vi "3Act Helper - DynamixelPositionAdjustment 0_360.vi"(10 "Dynamixel Setpoint In (deg)":dbl, 11 "Dynamixel Set Data":T1) -> (3 "Dynamixel Setpoint Out (deg)":dbl)   [LabVIEW 2013]
doc: "Because the Dynamixel is (theoretically) a 0-360 deg position controlled motor, we will need to only command 0-360 values, and keep track of the loop counts to find out where the motor really is. This really needs to be tested with the actual Dynamixels.\n\nEric Schneider, March 2014"
uses:
  Data/TypeDefs/DynamixelSetupInfo.ctl
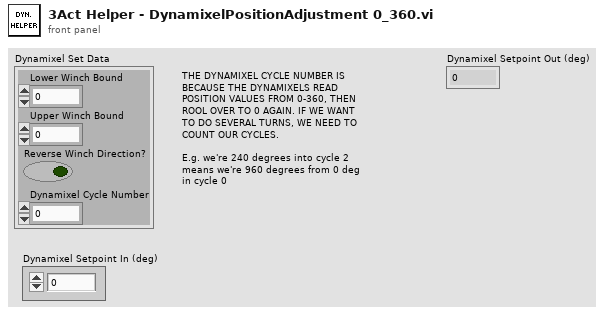
[diagram p1: front panel]
types:
  T1 = typedef "DynamixelSetupInfo.ctl" = cluster{"Lower Winch Bound":dbl, "Upper Winch Bound":dbl, "Reverse Winch Direction?":bool, "Dynamixel Cycle Number":i32}
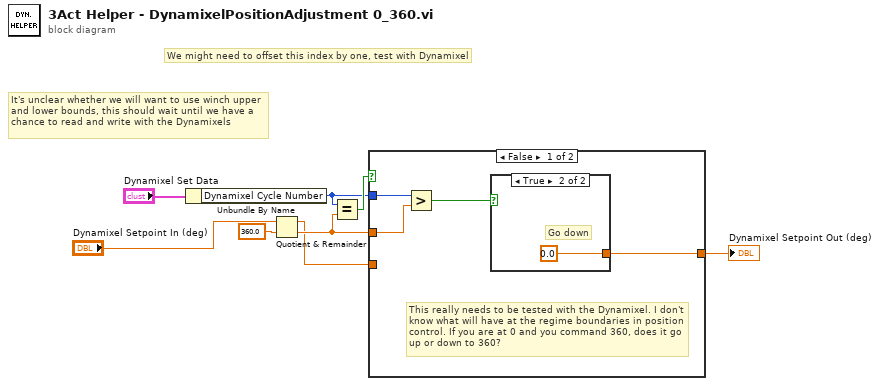
[diagram p0: block diagram]
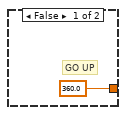
[diagram p2: hidden frame]
diagram:
  # "We might need to offset this index by one, test with Dynamixel"
  # "It's unclear whether we will want to use winch upper and lower bounds, this should wait until we have a chance to read and write with the Dynamixels"
  n1 = Unbundle By Name("Dynamixel Set Data") -> ("Dynamixel Cycle Number"=w3:i32)
  n2 = Quotient & Remainder(x="Dynamixel Setpoint In (deg)", y=360.0) -> (x-y*floor(x/y)=w1:dbl, floor(x/y)=w2:dbl)
  n3 = Equal?(x=w3, y=w2) -> (x = y?=w6:bool)
  n4 = case shown="False" w6 {
    tunnel: [w9 w15] -> w4
    tunnel: w1 -> [_ w15]
    tunnel: w3 -> [w12 _]
    tunnel: w2 -> [w11 _]
    frame False {
      # "This really needs to be tested with the Dynamixel. I don't know what will have at the regime boundaries in position control. If you are at 0 and you command 360, does it go up or down to 360?"
      n5 = Greater?(x=w12, y=w11) -> (0:w10:bool)
      n6 = case shown="True" w10 {
        tunnel: [360.0 ("y") 0.0 ("y")] -> w9
        frame False {
          # "GO UP"
        }
        frame True {
          # "Go down"
        }
      }
    }
    frame True {
    }
  }
  "Dynamixel Setpoint Out (deg)" <- w4
